vi "On Compile Action VI Name.vi"(11 "CD Template in":refnum<class "NIVS_PPL_Inline HW Interface.lvclass">) -> (2 "On Compile Action VI Name":string)   [LabVIEW 2020, in "NIVS_PPL_Inline HW Interface.lvclass"]
uses:
  NIVS_PPL_Inline HW Interface.lvclass
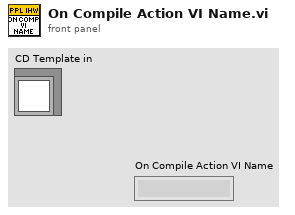
[diagram p1: front panel]
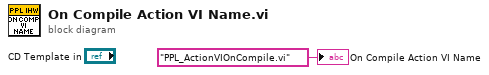
[diagram p0: block diagram]
diagram:
  "On Compile Action VI Name" <- "PPL_ActionVIOnCompile.vi" ("On Compile Action VI Name")
